vi "Write String from Control.vi"(8 "error in (no error)":errorcluster, 10 "String":string, 11 "Display Panel V3 in":refnum<class "Display Panel V3.lvclass">) -> (0 "error out":errorcluster, 3 "Display Panel V3 out":refnum<class "Display Panel V3.lvclass">)   [LabVIEW 2014, in "Display Panel.lvlib" / "Display Panel V3.lvclass"]
uses:
  Display Panel V3.lvclass
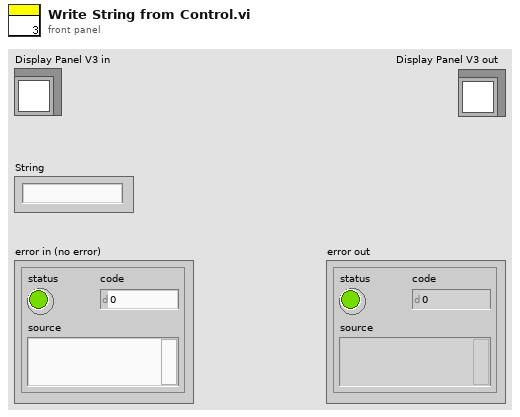
[diagram p1: front panel]
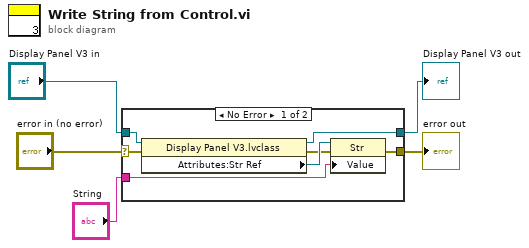
[diagram p0: block diagram]
diagram:
  n1 = case shown="No Error" "error in (no error)" {
    selector: "error in (no error)" -> [w8 w13]
    tunnel: [w7 w13] -> w4
    tunnel: "Display Panel V3 in" -> [w12 w14]
    tunnel: [w11 w14] -> w2
    tunnel: "String" -> [w6 _]
    frame No Error {
      n2 = property class="Display Panel V3.lvclass"(reference=w12, error in=w8) -> (reference out=w11:refnum<class "Display Panel V3.lvclass">, error out=w9:errorcluster, "Attributes:Str Ref"=w10:refnum<vi>)
      n3 = property class="Str"(reference=w10, error in=w9, "Value"=w6) -> (error out=w7:errorcluster)  [unwired: 1 out]
    }
    frame Error {
    }
  }
  "Display Panel V3 out" <- w2
  "error out" <- w4
